vi "CHROMA Set Voltage Range.vi"(8 "Error In":errorcluster, 9 "Voltage Limit":i32=130, 10 "Voltage Range":T1, 11 "CHROMA VISA In":refnum<visa-resource-name>) -> (0 "Error Out":errorcluster, 3 "CHROMA VISA Out":refnum<visa-resource-name>)   [LabVIEW 2019]
uses:
  Type Definition/CHROMA Voltage Range.ctl
  Type Definition/CHROMA Build CMD Type.ctl
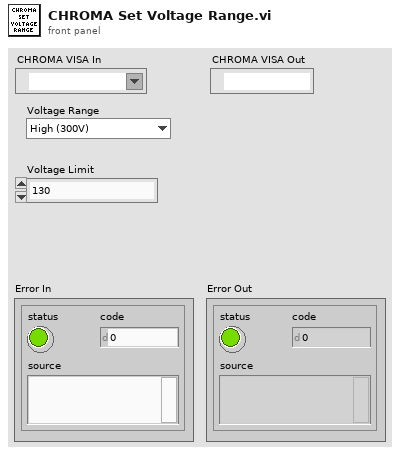
[diagram p1: front panel]
types:
  T1 = typedef "CHROMA Voltage Range.ctl" = enum16{"High (300V)", "Low (150V)"}
  T2 = typedef "CHROMA Build CMD Type.ctl" = enum16{"Value DBL", "Value I32", "String"}
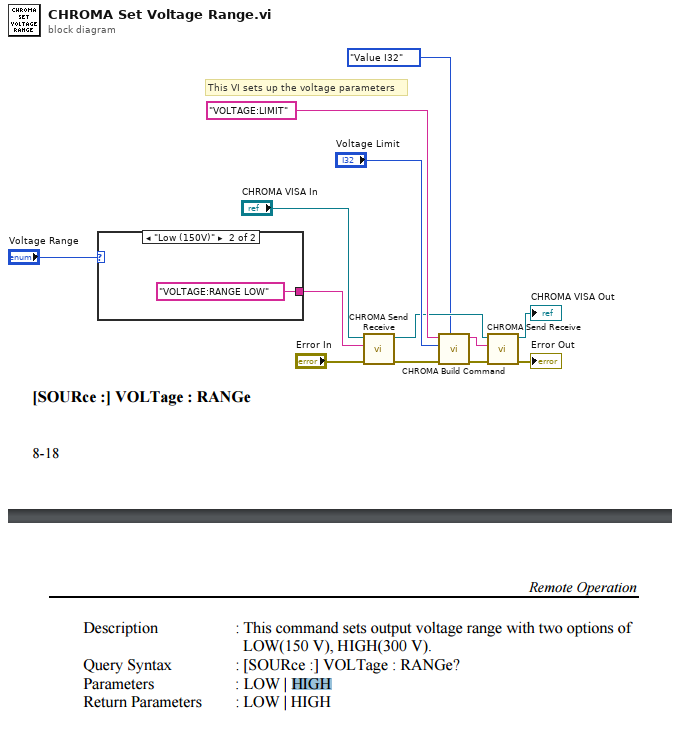
[diagram p0: block diagram]
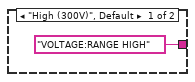
[diagram p2: hidden frame]
diagram:
  # "This VI sets up the voltage parameters"
  n1 = case shown="\"Low (150V)\"" "Voltage Range" {
    tunnel: ["VOLTAGE:RANGE HIGH" ("string to write") "VOLTAGE:RANGE LOW" ("string to write")] -> w9
    frame "High (300V)", Default {
    }
    frame "Low (150V)" {
    }
  }
  n2 = call "CHROMA Send Receive.vi"("error in (no error)"="Error In", "Send Command"=w9, "CHROMA VISA In"="CHROMA VISA In") -> ("error out"=w3:errorcluster, "CHROMA VISA Out"=w11:refnum<visa-resource-name>)  [unwired: 6 in, 1 out]
  n3 = call "CHROMA Build Command.vi"("Build Type"=CHROMA_Build_CMD_Type."Value I32", "Error In"=w3, "Value"="Voltage Limit", "Partial Command"="VOLTAGE:LIMIT" ("string to write")) -> ("Error Out"=w2:errorcluster, "Chroma Command"=w7:string)  [unwired: 6 in]
  n4 = call "CHROMA Send Receive.vi"("error in (no error)"=w2, "Send Command"=w7, "CHROMA VISA In"=w11) -> ("error out"=→"Error Out":errorcluster, "CHROMA VISA Out"=→"CHROMA VISA Out":refnum<visa-resource-name>)  [unwired: 6 in, 1 out]
